vi "Sub_Build_Variable_Header_Connect.vi"(8 "error in (no error)":errorcluster, 9 "Connect Flags":T1={"user name"=FALSE, "password"=FALSE, "will retain"=TRUE, "will flag"=FALSE, "clean session"=FALSE, "reserved"=FALSE, "will QoS"=enum."At most once"}, 10 "Keep Alive (sec)":u16) -> (0 "error out":errorcluster, 2 "Variable Header":u8[](array[numeric]) format="%x")   [LabVIEW 2013, in "MQTT_Functions.lvlib"]
uses:
  MQTT_Functions.lvlib
  Controls/Connect_Flags.ctl
  Controls/QoS.ctl
panel:
  in  "Protocol Name":string="MQTT"
  in  "Protocol Version":u8=4
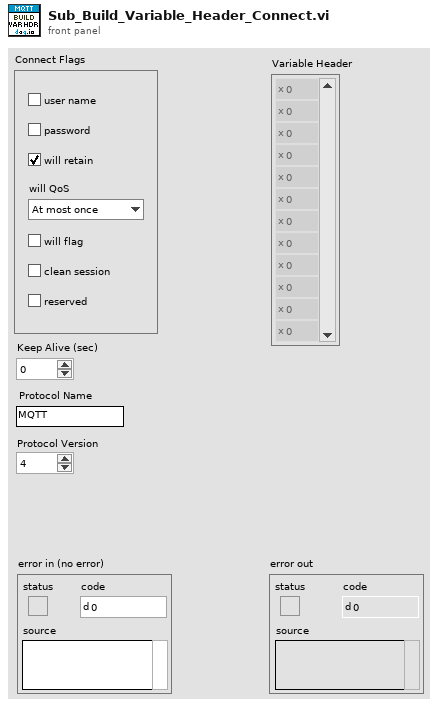
[diagram p1: front panel]
types:
  T1 = typedef "MQTT_Functions.lvlib/Connect_Flags.ctl" = cluster{"user name":bool, "password":bool, "will retain":bool, "will flag":bool, "clean session":bool, "reserved":bool, "will QoS":T2}
  T2 = typedef "MQTT_Functions.lvlib/QoS.ctl" = enum8{"At most once", "At least once", "Exactly once", "Reserved"}
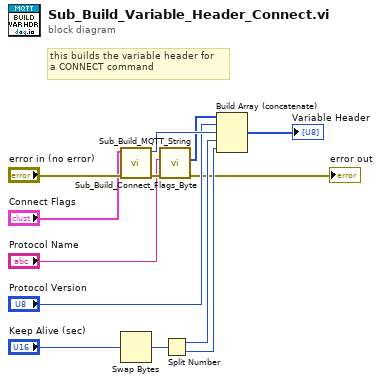
[diagram p0: block diagram]
diagram:
  # "this builds the variable header for \na CONNECT command"
  n1 = call "Sub_Build_Connect_Flags_Byte.vi"("error in (no error)"="error in (no error)", "Connect Flags"="Connect Flags") -> ("error out"=w4:errorcluster, "ConnectFlags Byte"=w10:u8)  [unwired: 8 in]
  n2 = Swap Bytes(anything="Keep Alive (sec)") -> (byte swapped=w11:u16)
  n3 = call "Sub_Build_MQTT_String.vi"("error in (no error)"=w4, "String to be encoded"="Protocol Name") -> ("error out"=→"error out":errorcluster, "UTF8 Byte Array"=w2:u8[])  [unwired: 8 in]
  n4 = Split Number(x=w11) -> (hi(x)=w9:u8, lo(x)=w8:u8)
  n5 = Build Array (concatenate)(w2, "Protocol Version", w10, w9, w8) -> (→"Variable Header":u8[])
